vi "Define Slew Rate.vi"(7 "Channel (0: Channel A)":u16(ring) items=["Channel A", "Channel B"], 8 "error in (no error)":errorcluster, 10 "Slew Rate (100)":dbl=100.0, 11 "BH Druck PACE Series in":refnum<class "BH Druck PACE Series.lvclass">) -> (0 "error out":errorcluster, 2 "Slew Rate Issued":dbl, 3 "BH Druck PACE Series out":refnum<class "BH Druck PACE Series.lvclass">)   [LabVIEW 2022 SP3, in "BH Druck PACE Series.lvclass"]
uses:
  BH Druck PACE Series.lvclass
  BH Druck PACE Series.lvclass/BH Druck PACE Series.ctl
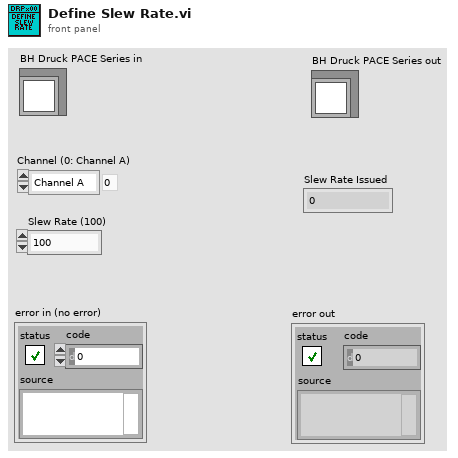
[diagram p1: front panel]
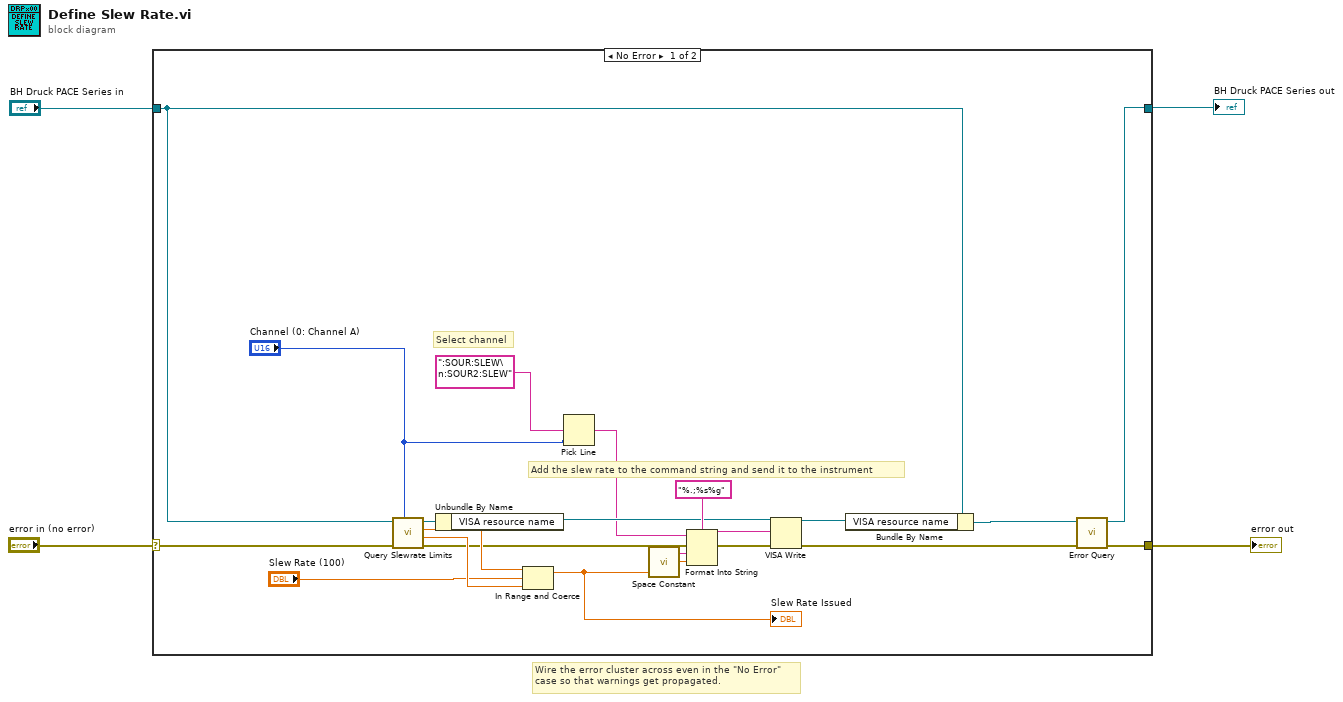
[diagram p0: block diagram]
diagram:
  # "Wire the error cluster across even in the \"No Error\"\ncase so that warnings get propagated."
  n1 = case shown="No Error" "error in (no error)" {
    selector: "error in (no error)" -> [w25 w27]
    tunnel: [w8 w27] -> w3
    tunnel: [w5 w26] -> w1
    tunnel: "BH Druck PACE Series in" -> [w13 w26]
    frame No Error {
      # "Add the slew rate to the command string and send it to the instrument"
      # "Select channel"
      n2 = call-dynamic "Query Slewrate Limits.vi"("Channel (0: Channel A)"="Channel (0: Channel A)", "error in (no error)"=w25, "BH Druck PACE Series in"=w13) -> ("error out"=w17:errorcluster, "Lower Slew Rate Limit"=w19:dbl, "Upper Slew Rate Limit"=w20:dbl, "BH Druck PACE Series out"=w16:refnum<class "BH Druck PACE Series.lvclass">)  [unwired: 5 in]
      n3 = Unbundle By Name(w16) -> ("VISA resource name"=w15:refnum<visa-resource-name>)
      n4 = In Range and Coerce(upper limit=w20, x="Slew Rate (100)", lower limit=w19) -> (coerced(x)=w14:dbl)  [unwired: 1 out]
      "Slew Rate Issued" <- w14
      n5 = Pick Line(multi-line string=":SOUR:SLEW\n:SOUR2:SLEW", line index="Channel (0: Channel A)") -> (output string=w11:string)  [unwired: 1 in]
      n6 = call <vilib>:"Space Constant.vi"() -> ("String"=w22:string)
      n7 = Format Into String(format string="%.;%s%g", initial string=w11, error in=w17, w22, w14) -> (resulting string=w24:string, error out=w23:errorcluster)
      n8 = VISA Write(VISA resource name=w15, write buffer=w24, error in (no error)=w23) -> (VISA resource name out=w12:refnum<visa-resource-name>, error out=w7:errorcluster)  [unwired: 1 out]
      n9 = Bundle By Name(cluster=w13, "VISA resource name"=w12) -> (w6:refnum<class "BH Druck PACE Series.lvclass">)
      n10 = call-dynamic "Error Query.vi"("error in (no error)"=w7, "BH Druck PACE Series in"=w6) -> ("error out"=w8:errorcluster, "BH Druck PACE Series out"=w5:refnum<class "BH Druck PACE Series.lvclass">)  [unwired: 8 in]
    }
    frame Error {
    }
  }
  "error out" <- w3
  "BH Druck PACE Series out" <- w1
